vi "HTTP parse headers.vi"(11 "HTTP headers":string="HTTP/1.1 409 Conflict\r\nAccess-Control-Allow-Headers: Origin, X-Requested-With, Content-Type, Accept\r\nAccess-Control-Allow-Methods: GET, POST, PUT, DELETE\r\nAccess-Control-Allow-Origin: *\r\nAccess-Control-Max-Age: 2592000\r\nContent-Type: text/plain\r\nX-Influxdb-Version: InfluxDB v0.8.8 (git: afde71e) (leveldb: 1.15)\r\nDate: Thu, 23 Apr 2015 18:50:38 GMT\r\nContent-Length: 21\r\n\r\n") -> (0 "Headers out":T1, 1 "Status":string, 2 "Status code":string, 3 "HTTP version":string)   [LabVIEW 2018]
doc: "Parse HTTP headers to retrieve status information."
uses:
  <userlib>/_OpenG.lib/dictionary/dictionary.llb/Dictionary Object RefNum__ogtk.ctl
  <userlib>/_OpenG.lib/dictionary/dictionary.llb/Dictionary Object RefNum - Enum__ogtk.ctl
  <userlib>/_OpenG.lib/dictionary/dictionary.llb/Dictionary Update (by scalar value)__ogtk.vi
  <vilib>/regexp/Match Regular Expression.xnode
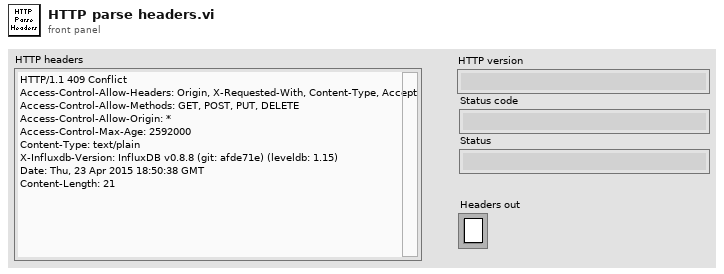
[diagram p1: front panel]
types:
  T1 = typedef "Dictionary Object RefNum__ogtk.ctl" = refnum<k1>
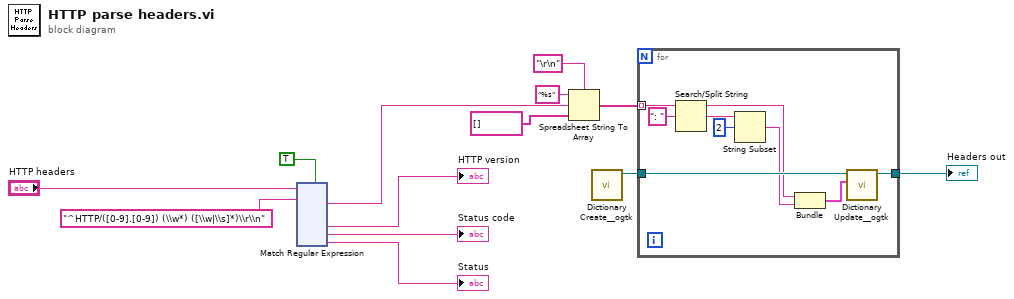
[diagram p0: block diagram]
diagram:
  n1 = xnode "Match Regular Expression"("input string"="HTTP headers", "regular expression"="^HTTP/([0-9].[0-9]) (\\w*) ([\\w|\\s]*)\\r\\n", "multiline? (F)"=TRUE) -> ("after match"=w1:string, "submatch 1"=→"HTTP version":string, "submatch 2"=→"Status code":string, "submatch 3"=→"Status":string)  [unwired: 3 in, 4 out]
  n2 = Spreadsheet String To Array(delimiter (Tab)="\r\n", format string="%s", spreadsheet string=w1, array type (2D Dbl)=string[] []) -> (array=w5:string[])
  n3 = call <userlib>:"Dictionary Create__ogtk.vi"() -> ("dictionary out"=w4:T1)  [unwired: 10 in, 1 out]
  n4 = for {
    tunnel: w5 -> [w22] mode=indexing
    tunnel: w4 -> [w18]
    tunnel: [w14] -> w3
    n5 = Search/Split String(string=w22, search string/char (-)=": ") -> (substring before match=w17:string, match + rest of string=w19:string)  [unwired: 1 in, 1 out]
    n6 = String Subset(string=w19, offset (0)=2) -> (substring=w16:string)  [unwired: 1 in]
    n7 = Bundle(w17, w16) -> (w15:cluster{string, string})  [unwired: 1 in]
    n8 = call-poly <userlib>:"Dictionary Update__ogtk.vi"("key-value"=w15, "dictionary"=w18) -> ("dictionary out"=w14:T1)  [unwired: 7 in, 2 out]
  }
  "Headers out" <- w3
